vi "InlineCNodeAddIO.vi"(0 "__args":T1) -> (1 "__return":i32, 2 "__errStatus":bool, 3 "__errCode":i32, 4 "__errSource":string)   [LabVIEW 2013]
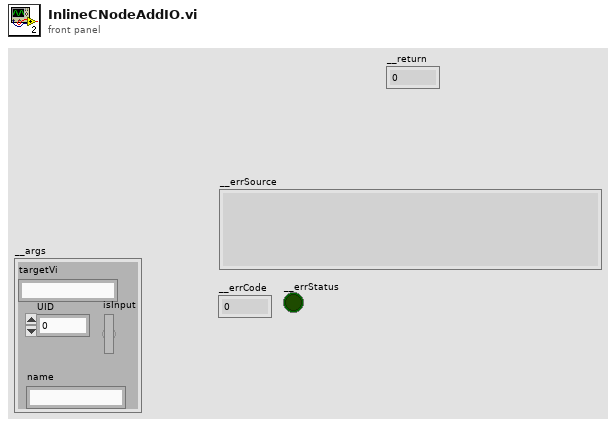
[diagram p1: front panel]
types:
  T1 = cluster{"targetVi":string, "UID":i32, "isInput":bool, "name":string}
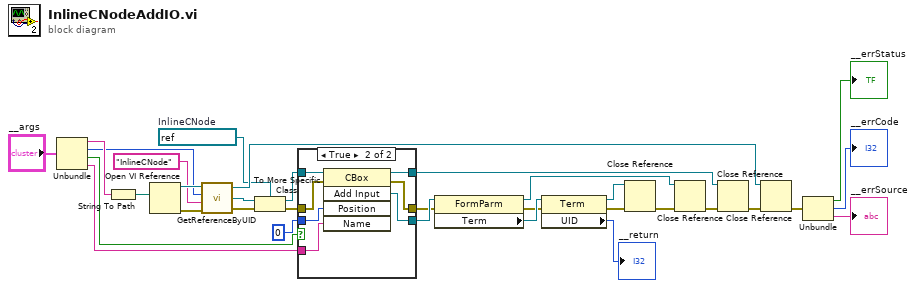
[diagram p0: block diagram]
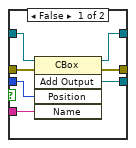
[diagram p2: hidden frame]
diagram:
  w15 = refnum<vi> refnum  # InlineCNode
  n1 = Unbundle("__args") -> ("targetVi"=w26:string, "UID"=w24:i32, "isInput"=w18:bool, "name"=w16:string)
  n2 = String To Path(string=w26) -> (path=w28:path)
  n3 = Open VI Reference(vi path=w28) -> (vi reference=w25:refnum<vi>, error out=w27:errorcluster)  [unwired: 5 in]
  n4 = call "GetReferenceByUID.vi"("error in (no error)"=w27, "objectClass"="InlineCNode", "UID"=w24, "targetVI"=w25) -> ("error out"=w23:errorcluster, "refNum"=w22:refnum<vi>, "dup targetVI"=w21:refnum<vi>)
  n5 = To More Specific Class(target class=w15, reference=w22, error in=w23) -> (specific class reference=w20:refnum<vi>, error out=w19:errorcluster)
  n6 = case shown="True" w18 {
    tunnel: w20 -> [w39 w46]
    tunnel: w19 -> [w38 w45]
    tunnel: [w37 w43] -> w17
    tunnel: w16 -> [w36 w44]
    tunnel: [w34 w42] -> w13
    tunnel: [w35 w41] -> w7
    tunnel: u32 0 ("Position") -> [w33 w40]
    frame False {
      n7 = invoke class="CBox" method="Add Output"(reference=w39, error in=w38, "Position"=w33, "Name"=w36) -> (reference out=w37:refnum<vi>, error out=w35:errorcluster, "Add Output"=w34:refnum<vi>)  [unwired: 1 in, 2 out]
    }
    frame True {
      n8 = invoke class="CBox" method="Add Input"(reference=w46, error in=w45, "Position"=w40, "Name"=w44) -> (reference out=w43:refnum<vi>, error out=w41:errorcluster, "Add Input"=w42:refnum<vi>)  [unwired: 1 in, 2 out]
    }
  }
  n9 = property class="FormParm"(reference=w13, error in=w7) -> (reference out=w1:refnum<vi>, error out=w6:errorcluster, "Term"=w9:refnum<vi>)
  n10 = property class="Term"(reference=w9, error in=w6) -> (reference out=w2:refnum<vi>, error out=w3:errorcluster, "UID"=→"__return":i32)
  n11 = Close Reference(reference=w2, error in (no error)=w3) -> (error out=w5:errorcluster)
  n12 = Close Reference(reference=w1, error in (no error)=w5) -> (error out=w4:errorcluster)
  n13 = Close Reference(reference=w17, error in (no error)=w4) -> (error out=w11:errorcluster)
  n14 = Close Reference(reference=w21, error in (no error)=w11) -> (error out=w12:errorcluster)
  n15 = Unbundle(w12) -> ("status"=→"__errStatus":bool, "code"=→"__errCode":i32, "source"=→"__errSource":string)
